vi "control-a-pwm-frec.vi"() -> ()   [LabVIEW 2013]
uses:
  <vilib>/MakerHub/LINX/Public/Utilities/Open Serial.vi
  <instrlib>/RIGOL DS1000 Series/Public/Configure/Configure Trigger (Edge).vi
  <vilib>/MakerHub/LINX/LMH-LINX.lvlib
  <instrlib>/RIGOL DS1000 Series/RIGOL DS1000 Series.lvlib
  <vilib>/Analysis/NI_AALBase.lvlib
panel:
  in  "Tab Control":enum32{"CONTROLES", "GRAFICA"}(tab)
  in  "stop 2":bool
  in  "Arduino Port":refnum<visa-resource-name>="N/A"
  in  "stop":bool
  in  "PWM":dbl(knob)=10.0 min=10.0 max=90.0 step=1.0 scale=10.0..90.0 scale format="%#_2g"
  out "PWM Apagado":cluster{"Y":dbl[], "Y":dbl[]}[](graph)
  out "Loop Rate (Hz)":u32
  out "RPM 2":dbl
  in  "Osc Port":refnum<visa-resource-name>="N/A"
  out "RPM":dbl(knob) scale=-5000.0..5000.0
  out "encendido":bool
  out "apagado":bool
  in  "FRECUENCIA":u16(slide) scale=0.0..15000.0
  out "PWM VS RPM":cluster{"Y":dbl[], "Y":dbl[]}[](graph)
  # "rpm"
  # "Hz"
  # "IZQUIERDA"
  # "DERECHA"
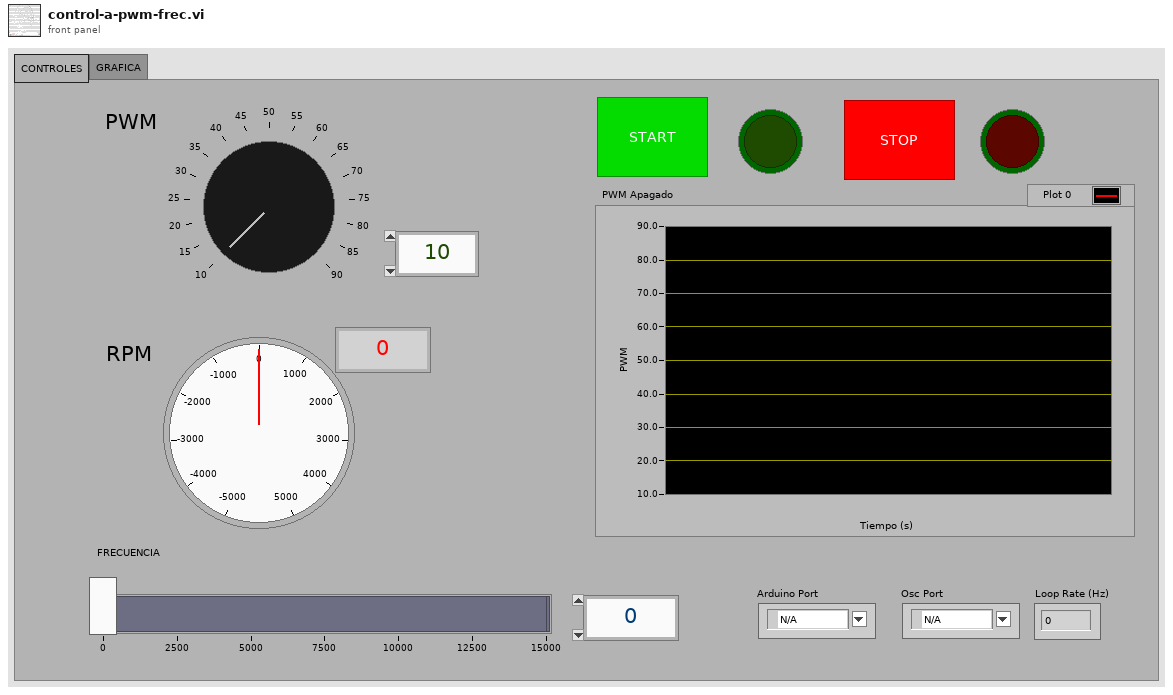
[diagram p1: front panel]
types:
  T1 = typedef "LMH-LINX.lvlib/LINX Ref.ctl" = cluster{"IO":T2, "Interface":T3, "LINX Device Config":T4}
  T2 = typedef "LMH-LINX.lvlib/Platform.ctl" = enum16{"Remote", "Local"}
  T3 = typedef "LMH-LINX.lvlib/Interface.ctl" = enum16{"Serial", "TCP"}
  T4 = typedef "LMH-LINX.lvlib/Device.lvlib/LINX Device Config.ctl" = cluster{"Interface":T3, "COM Port":refnum<visa-resource-name>, "TCP Configuration":T5, "Device Family":u8, "Device ID":u8, "Device Name":string, "TCP Ref":refnum<k5>, "Channels":T6}
  T5 = typedef "LMH-LINX.lvlib/Device.lvlib/TCP Config.ctl" = cluster{"IP Address":string, "Port":u16}
  T6 = typedef "LMH-LINX.lvlib/Channels.ctl" = cluster{"DI":u8[], "DO":u8[], "AI":u8[], "AO":u8[], "PWM":u8[], "QE":u8[], "UART":u8[], "I2C 2":u8[], "SPI":u8[], "CAN":u8[], "Servo":u8[], "AI Ref (V)":dbl, "AI Resolution (Bits)":u8, "AO Ref (V)":dbl, "AO Resolution (Bits)":u8}
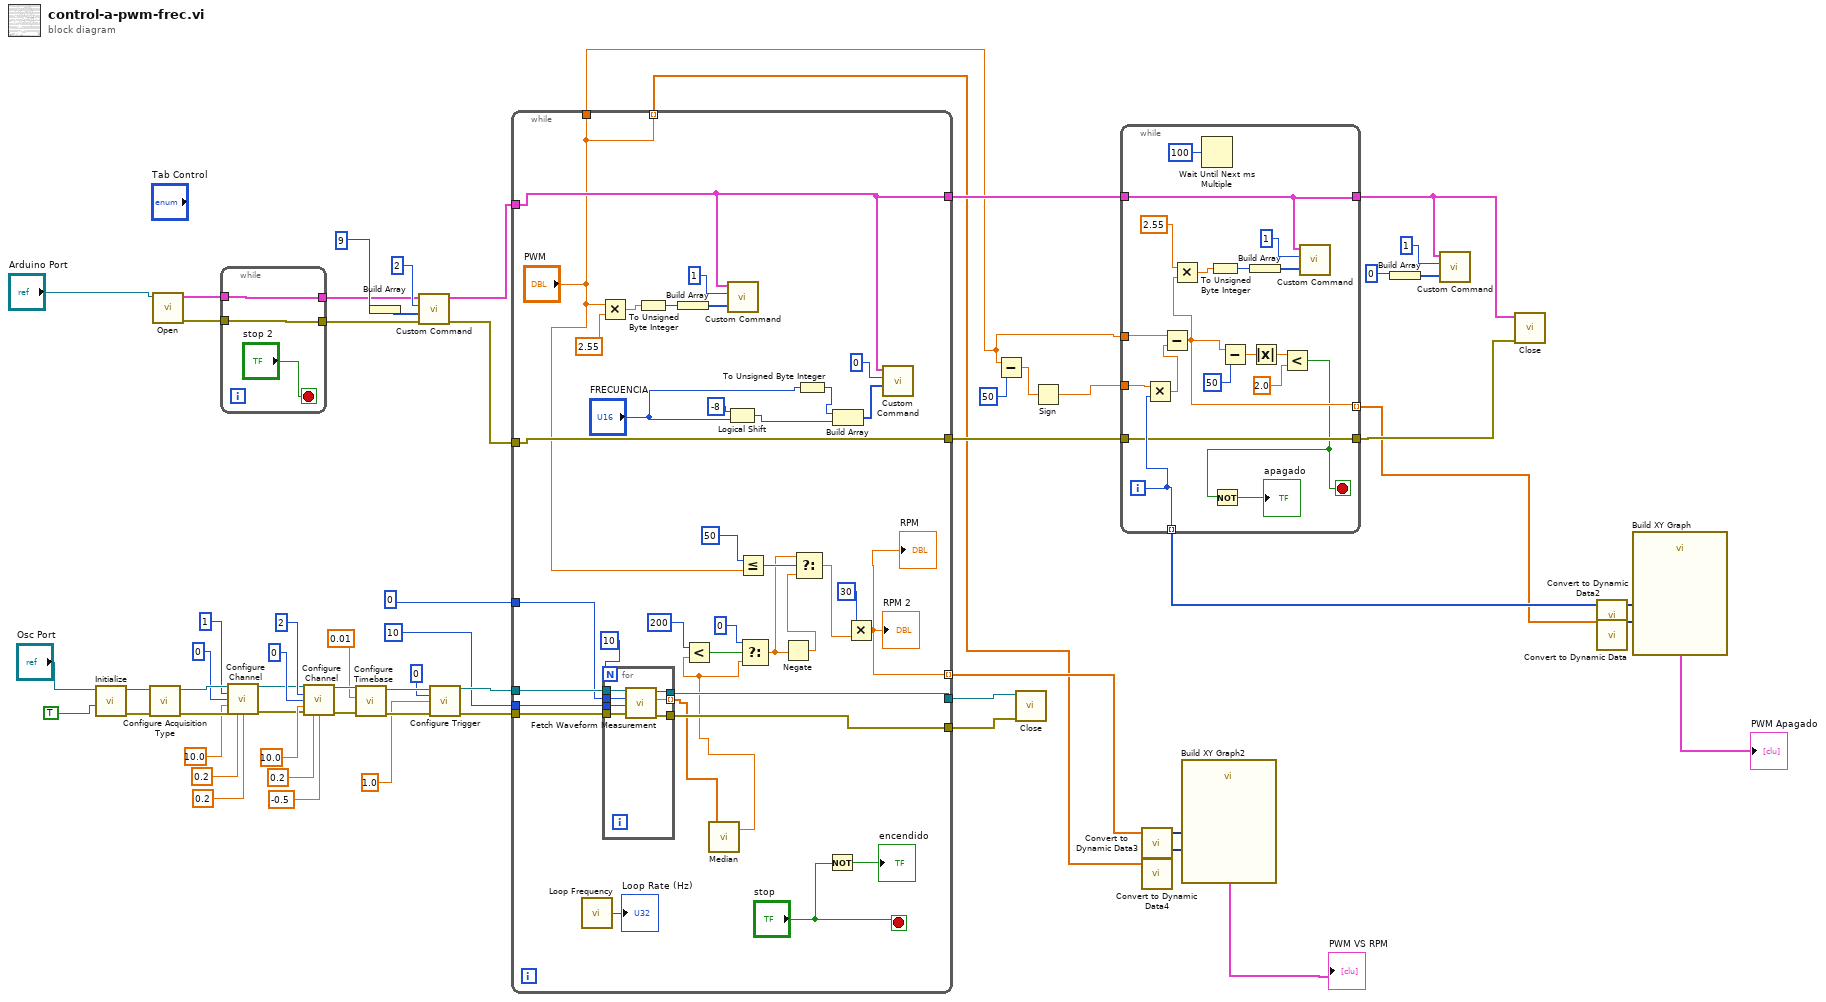
[diagram p0: block diagram]
diagram:
  n1 = call <instrlib>:"Initialize.vi"("Reset (True)"=TRUE, "VISA resource name"="Osc Port") -> ("error out"=w40:errorcluster, "VISA resource name out"=w39:refnum<visa-resource-name>)  [unwired: 8 in]
  n2 = call <instrlib>:"Configure Acquisition Type.vi"("error in (no error)"=w40, "VISA resource name"=w39) -> ("error out"=w37:errorcluster, "VISA resource name out"=w38:refnum<visa-resource-name>)  [unwired: 8 in]
  n3 = call-poly <vilib>:"Open.vi"("Serial Port"="Arduino Port") -> ("Error Out"=w1:errorcluster, "LINX Resource"=w3:T1)  [unwired: 8 in, 1 out]
  n4 = while {
    tunnel: [w64] -> w4
    tunnel: w3 -> [w64]
    tunnel: [w63] -> w2
    tunnel: w1 -> [w63]
    stop <- "stop 2" stop-if-true
  }
  n5 = call <instrlib>:"Configure Channel.vi"("VISA resource name"=w38, "Channel (1: Channel 1)"=1, "Vertical Coupling (0: DC)"=0, "Probe Attenuation (1.0)"=10.0, "error in (no error)"=w37, "Vertical Range (1.0 V)"=0.2, "Vertical Offset (0.0 V)"=0.2) -> ("VISA resource name out"=w27:refnum<visa-resource-name>, "error out"=w26:errorcluster)  [unwired: 7 in]
  n6 = call <instrlib>:"Configure Channel.vi"("VISA resource name"=w27, "Channel (1: Channel 1)"=2, "Vertical Coupling (0: DC)"=0, "Probe Attenuation (1.0)"=10.0, "error in (no error)"=w26, "Vertical Range (1.0 V)"=0.2, "Vertical Offset (0.0 V)"=-0.5) -> ("VISA resource name out"=w23:refnum<visa-resource-name>, "error out"=w24:errorcluster)  [unwired: 7 in]
  n7 = call <instrlib>:"Configure Timebase.vi"("error in (no error)"=w24, "Timebase (0.0005 s)"=0.01, "VISA resource name"=w23) -> ("error out"=w20:errorcluster, "VISA resource name out"=w21:refnum<visa-resource-name>)  [unwired: 7 in]
  n8 = Build Array(9) -> (w60:i32[])
  n9 = call <vilib>:"Custom Command.vi"("Error In"=w2, "Data"=w60, "Custom Command Number"=2, "LINX Resource"=w4) -> ("Error Out"=w62:errorcluster, "LINX Resource"=w43:T1)  [unwired: 4 in, 2 out]
  n10 = call-poly <instrlib>:"Configure Trigger.vi"("VISA resource name"=w21, "Trigger Source (0: Channel 1)"=0, "Trigger Level (0.0 V)"=1.0, "error in (no error)"=w20) -> ("VISA resource name out"=w15:refnum<visa-resource-name>, "error out"=w14:errorcluster)  [unwired: 10 in]
  n11 = while {
    tunnel: w43 -> [w89]
    tunnel: w62 -> [w101]
    tunnel: [w89] -> w53
    tunnel: [w101] -> w48
    tunnel: ["PWM"] -> w51
    tunnel: [w87] -> w17
    tunnel: [w86] -> w16
    tunnel: w15 -> [w85]
    tunnel: w14 -> [w84]
    tunnel: 10 -> [w83]
    tunnel: 0 -> [w82]
    tunnel: [w80] -> w9 mode=indexing
    tunnel: ["PWM"] -> w8 mode=indexing
    stop <- "stop" stop-if-true
    n12 = call <vilib>:"Loop Frequency.vi"() -> ("Loop Rate (Hz)"=→"Loop Rate (Hz)":u32)
    n13 = Multiply(x="PWM", y=2.55) -> (x*y=w94:dbl)
    n14 = for {
      N: 10 -> [_]
      tunnel: [w108] -> w87
      tunnel: [w107] -> w86
      tunnel: w85 -> [w106]
      tunnel: w84 -> [w105]
      tunnel: w83 -> [w104]
      tunnel: w82 -> [w103]
      tunnel: [w102] -> w68 mode=indexing
      n15 = call <instrlib>:"Fetch Waveform Measurement.vi"("error in (no error)"=w105, "Measurement Function (0: Voltage Vpp)"=w104, "Source (0: Channel 1)"=w103, "VISA resource name"=w106) -> ("error out"=w108:errorcluster, "Measured Value"=w102:dbl, "VISA resource name out"=w107:refnum<visa-resource-name>)  [unwired: 5 in]
    }
    n16 = To Unsigned Byte Integer(number=w94) -> (unsigned 8bit integer=w95:u8)
    n17 = Build Array(w95) -> (w98:u8[])
    n18 = call <vilib>:"Median.vi"("X"=w68) -> ("median"=w66:dbl)  [unwired: 1 out]
    n19 = Less?(x=200, y=w66) -> (x < y?=w78:bool)
    n20 = Logical Shift(y=-8, x="FRECUENCIA") -> (x << y=w91:u16)
    n21 = call <vilib>:"Custom Command.vi"("Data"=w98, "Custom Command Number"=1, "LINX Resource"=w89) -> ()  [unwired: 5 in, 4 out]
    n22 = Less Or Equal?(x=50, y="PWM") -> (x <= y?=w75:bool)
    n23 = Select(t=0, s=w78, f=w66) -> (s? t:f=w72:dbl)
    n24 = Negate(x=w72) -> (-x=w71:dbl)
    n25 = Select(t=w72, s=w75, f=w71) -> (s? t:f=w73:dbl)
    n26 = To Unsigned Byte Integer(number="FRECUENCIA") -> (unsigned 8bit integer=w97:u8)
    n27 = Not(x="stop") -> (.not. x?=→"encendido":bool)
    n28 = Build Array(w97, w91) -> (w96:u16[])
    n29 = Multiply(x=30, y=w73) -> (x*y=w80:dbl)
    "RPM 2" <- w80
    "RPM" <- w80
    n30 = call <vilib>:"Custom Command.vi"("Data"=w96, "Custom Command Number"=0, "LINX Resource"=w89) -> ()  [unwired: 5 in, 4 out]
  }
  n31 = Subtract(x=w51, y=50) -> (x-y=w54:dbl)
  n32 = call <vilib>:"Close.vi"("error in (no error)"=w17, "VISA resource name"=w16) -> ()  [unwired: 9 in, 1 out]
  n33 = Sign(1:w54) -> (0:w50:dbl)
  n34 = while {
    tunnel: w53 -> [w120]
    tunnel: [w120] -> w52
    tunnel: w51 -> [w119]
    tunnel: w50 -> [w118]
    tunnel: [w117] -> w49 mode=indexing
    tunnel: w48 -> [w116]
    tunnel: [w116] -> w47
    tunnel: [w114] -> w46 mode=indexing
    i -> [w117]
    stop <- w109 stop-if-true
    n35 = Multiply(x=w118, y=w117) -> (x*y=w127:dbl)
    n36 = Subtract(x=w119, y=w127) -> (x-y=w114:dbl)
    n37 = Multiply(x=2.55, y=w114) -> (x*y=w122:dbl)
    n38 = Wait Until Next ms Multiple(millisecond multiple=u32 100) -> ()  [unwired: 1 out]
    n39 = To Unsigned Byte Integer(number=w122) -> (unsigned 8bit integer=w123:u8)
    n40 = Subtract(x=w114, y=50) -> (x-y=w113:dbl)
    n41 = Build Array(w123) -> (w124:u8[])
    n42 = Absolute Value(x=w113) -> (abs(x)=w112:dbl)
    n43 = Less?(x=w112, y=2.0) -> (x < y?=w109:bool)
    n44 = Not(x=w109) -> (.not. x?=→"apagado":bool)
    n45 = call <vilib>:"Custom Command.vi"("Data"=w124, "Custom Command Number"=1, "LINX Resource"=w120) -> ()  [unwired: 5 in, 4 out]
  }
  n46 = call "Convert to Dynamic Data3"("Array"=w9) -> ("Dynamic Data Type"=w11:dynamicdata)  [unwired: 3 in]
  n47 = call "Convert to Dynamic Data4"("Array"=w8) -> ("Dynamic Data Type"=w10:dynamicdata)  [unwired: 3 in]
  n48 = call "Build XY Graph2"("Y Input"=w11, "X Input"=w10) -> ("XY Graph"=→"PWM VS RPM":cluster{"X":dbl[], "Y":dbl[]}[])  [unwired: 8 in, 1 out]
  n49 = Build Array(0) -> (w56:i32[])
  n50 = call <vilib>:"Custom Command.vi"("Data"=w56, "Custom Command Number"=1, "LINX Resource"=w52) -> ()  [unwired: 5 in, 4 out]
  n51 = call <vilib>:"Close.vi"("Error In"=w47, "LINX Resource"=w52) -> ()  [unwired: 9 in, 1 out]
  n52 = call "Convert to Dynamic Data2"("Array"=w49) -> ("Dynamic Data Type"=w44:dynamicdata)  [unwired: 3 in]
  n53 = call "Convert to Dynamic Data"("Array"=w46) -> ("Dynamic Data Type"=w45:dynamicdata)  [unwired: 3 in]
  n54 = call "Build XY Graph"("Y Input"=w45, "X Input"=w44) -> ("XY Graph"=→"PWM Apagado":cluster{"X":dbl[], "Y":dbl[]}[])  [unwired: 8 in, 1 out]
